vi "Manual Intake Loop.vi"(9 "Gear IR":bool) -> (2 "Gear Piston Down?":bool, 3 "Roller Speed":dbl)   [LabVIEW 2016]
uses:
  Robot Global Data.vi
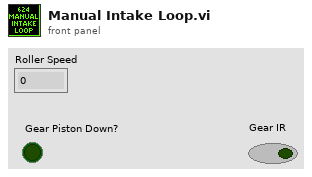
[diagram p1: front panel]
types:
  T1 = typedef "Manual Intake Control.ctl" = cluster{"Ball Intake/Outake":dbl, "Gear Intake/Outake":dbl}
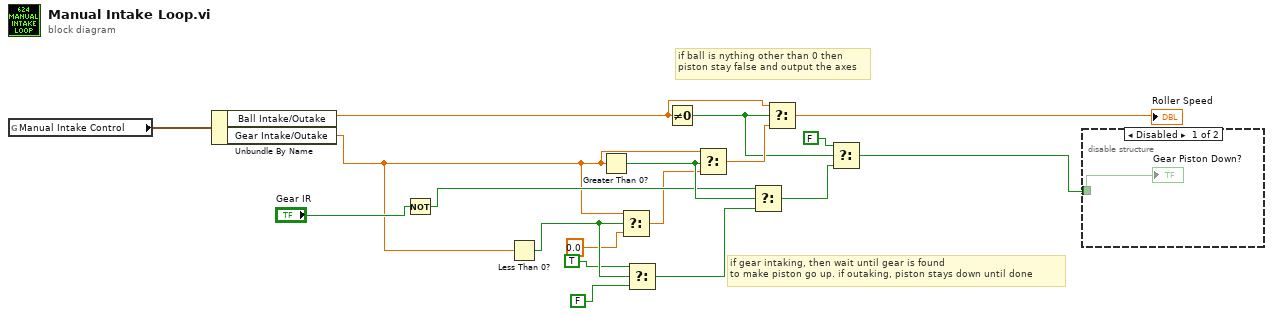
[diagram p0: block diagram]
diagram:
  # "if ball is nything other than 0 then \npiston stay false and output the axes"
  # "if gear intaking, then wait until gear is found\nto make piston go up. if outaking, piston stays down until done"
  n1 = global read "Robot Global Data.vi" "Manual Intake Control"() -> (w18:T1)
  n2 = Unbundle By Name(w18) -> ("Ball Intake/Outake"=w17:dbl, "Gear Intake/Outake"=w8:dbl)
  n3 = Not(x="Gear IR") -> (.not. x?=w10:bool)
  n4 = Less Than 0?(x=w8) -> (x < 0?=w7:bool)
  n5 = Greater Than 0?(x=w8) -> (x > 0?=w13:bool)
  n6 = Select(t=w8, s=w7, f=0.0) -> (s? t:f=w9:dbl)
  n7 = Select(t=TRUE, s=w7, f=FALSE) -> (s? t:f=w5:bool)
  n8 = Not Equal To 0?(x=w17) -> (x != 0?=w15:bool)
  n9 = Select(t=w8, s=w13, f=w9) -> (s? t:f=w16:dbl)
  n10 = Select(t=w10, s=w13, f=w5) -> (s? t:f=w12:bool)
  n11 = Select(t=w17, s=w15, f=w16) -> (s? t:f=→"Roller Speed":dbl)
  n12 = Select(t=FALSE, s=w15, f=w12) -> (s? t:f=w2:bool)
  n13 = disable-structure shown="Disabled" {
    disable-tunnel: w2 -> [w19 _]
    frame Disabled {
      "Gear Piston Down?" <- w19
    }
    frame Enabled {
    }
  }
